vi "New Terminal Binding.vi"(10 "Ctl Refnum":refnum<vi>) -> (0 "error out":errorcluster, 3 "TerminalBinding":refnum<class "TerminalBinding.lvclass">)   [LabVIEW 2017, in "Transport.lvlib" / "TerminalBinding.lvclass"]
doc: "<License>\nCopyright © 2017 Composed Systems, LLC | All rights reserved\nwww.composed.io\n\nAuthor: Ethan Stern <ethan.stern@composed.io>\n\nThis software is provided \"AS IS\" WITHOUT WARRANTIES, either express or implied, AND IS FOR EDUCATIONAL PURPOSES ONLY.\n</License>"
uses:
  TerminalBinding.lvclass
  TerminalBinding.lvclass/TerminalBinding.ctl
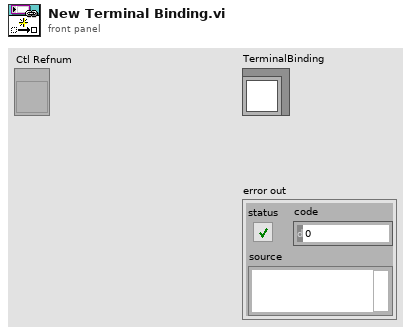
[diagram p1: front panel]
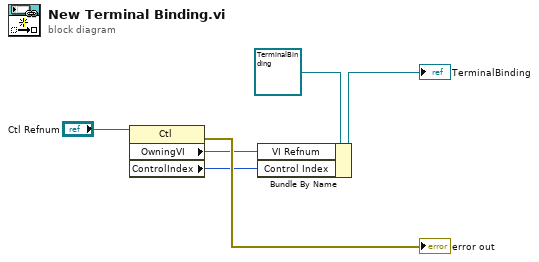
[diagram p0: block diagram]
diagram:
  n1 = property class="Ctl"(reference="Ctl Refnum") -> (error out=→"error out":errorcluster, "OwningVI"=w2:refnum<vi>, "ControlIndex"=w1:i32)  [unwired: 1 in, 1 out]
  n2 = Bundle By Name(cluster=refnum<class "TerminalBinding.lvclass"> refnum ("TerminalBinding in"), "VI Refnum"=w2, "Control Index"=w1) -> (→"TerminalBinding":refnum<class "TerminalBinding.lvclass">)
